vi "Or16.vi"(4 "b":bool[](array[boolean]), 5 "a":bool[](array[boolean])) -> (1 "out":bool[](array[boolean]))   [LabVIEW 2014]
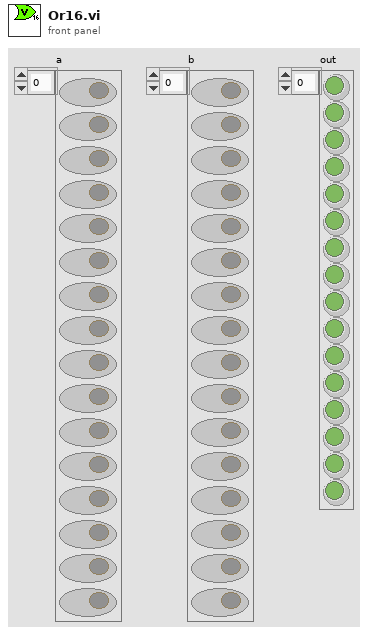
[diagram p1: front panel]
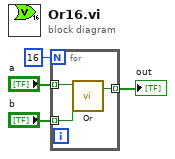
[diagram p0: block diagram]
diagram:
  n1 = for {
    N: 16 -> [_]
    tunnel: "a" -> [w7] mode=indexing
    tunnel: "b" -> [w6] mode=indexing
    tunnel: [w5] -> w1 mode=indexing
    n2 = call "Or.vi"("b"=w6, "a"=w7) -> ("out"=w5:bool)  [unwired: 3 in]
  }
  "out" <- w1
